vi "Log in and Post.vi"() -> ()   [LabVIEW 2019]
uses:
  firebase.lvclass
panel:
  in  "Data":T1 {"Dial" scale=0.0..10.0}
  in  "endPoint":string
  out "firebase out":refnum<class "firebase.lvclass">
  in  "Email":string
  in  "Password":string
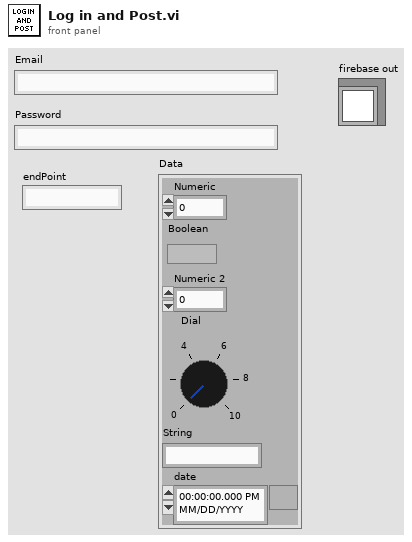
[diagram p1: front panel]
types:
  T1 = cluster{"Numeric":dbl, "Boolean":bool, "Numeric 2":dbl, "Dial":dbl, "String":string, "date":timestamp}
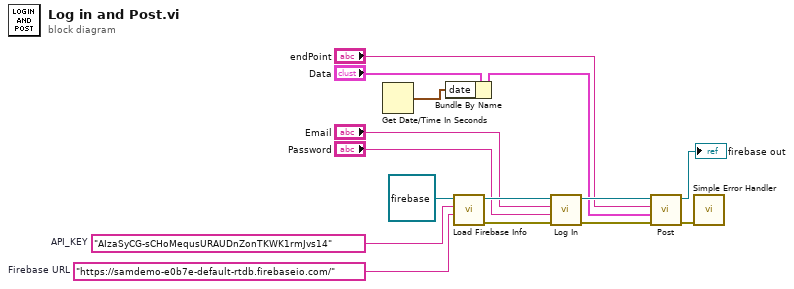
[diagram p0: block diagram]
diagram:
  w3 = "AIzaSyCG-sCHoMequsURAUDnZonTKWK1rmJvs14"  # API_KEY
  w4 = "https://samdemo-e0b7e-default-rtdb.firebaseio.com/"  # Firebase URL
  n1 = Get Date/Time In Seconds() -> (seconds since 1Jan1904=w1:timestamp)
  n2 = Bundle By Name(cluster="Data", "date"=w1) -> (w2:T1)
  n3 = call "Load Firebase Info.vi"("Firebase URL"=w4, "API_KEY"=w3, "firebase in"=refnum<class "firebase.lvclass"> refnum ("firebase.lvclass")) -> ("error out"=w15:errorcluster, "firebase out"=w11:refnum<class "firebase.lvclass">)  [unwired: 7 in]
  n4 = call-dynamic "Log In.vi"("error in"=w15, "password"="Password", "email"="Email", "firebase in"=w11) -> ("error out"=w14:errorcluster, "firebase out"=w8:refnum<class "firebase.lvclass">)  [unwired: 6 in]
  n5 = call-dynamic "Post.vi"("error in"=w14, "Anything"=w2, "endPoint"="endPoint", "firebase in"=w8) -> ("error out"=w13:errorcluster, "firebase out"=→"firebase out":refnum<class "firebase.lvclass">)  [unwired: 5 in, 1 out]
  n6 = call <vilib>:"Simple Error Handler.vi"("error in (no error)"=w13) -> ()  [unwired: 4 in, 5 out]
